vi "Shortest Distance Relative.vi"(10 "Needed angle":dbl(knob) scale=0.0..360.0, 11 "Current Angle":dbl(knob) scale=0.0..360.0) -> (2 "Flip motors?":bool, 3 "Degrees to travel":dbl)   [LabVIEW 2011, in "Pivot Drive.lvlib"]
uses:
  Pivot Drive.lvlib
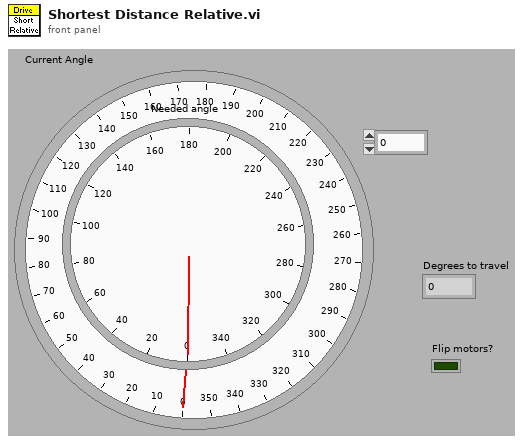
[diagram p1: front panel]
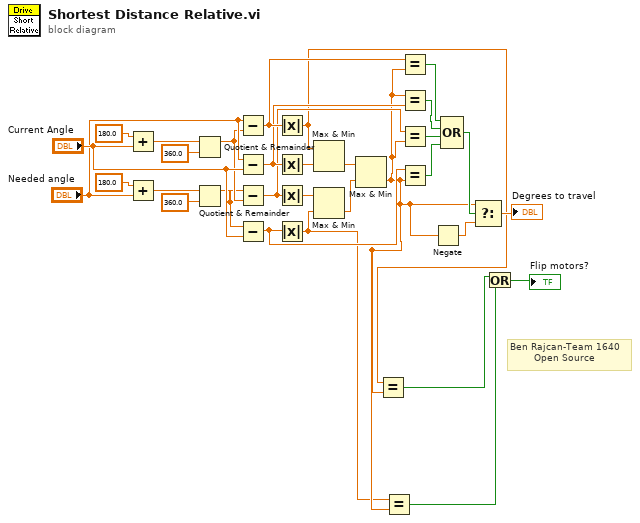
[diagram p0: block diagram]
diagram:
  # "Ben Rajcan-Team 1640\n        Open Source"
  n1 = Add(x=180.0, y="Current Angle") -> (x+y=w24:dbl)
  n2 = Add(x=180.0, y="Needed angle") -> (x+y=w27:dbl)
  n3 = Quotient & Remainder(x=w24, y=360.0) -> (x-y*floor(x/y)=w23:dbl)  [unwired: 1 out]
  n4 = Quotient & Remainder(x=w27, y=360.0) -> (x-y*floor(x/y)=w16:dbl)  [unwired: 1 out]
  n5 = Subtract(x="Needed angle", y=w23) -> (x-y=w11:dbl)
  n6 = Subtract(x="Needed angle", y="Current Angle") -> (x-y=w10:dbl)
  n7 = Subtract(x=w16, y=w23) -> (x-y=w9:dbl)
  n8 = Subtract(x=w16, y="Current Angle") -> (x-y=w8:dbl)
  n9 = Absolute Value(x=w11) -> (abs(x)=w4:dbl)
  n10 = Absolute Value(x=w10) -> (abs(x)=w3:dbl)
  n11 = Absolute Value(x=w9) -> (abs(x)=w2:dbl)
  n12 = Absolute Value(x=w8) -> (abs(x)=w1:dbl)
  n13 = Max & Min(x=w4, y=w3) -> (min(x,y)=w21:dbl)  [unwired: 1 out]
  n14 = Max & Min(x=w2, y=w1) -> (min(x,y)=w22:dbl)  [unwired: 1 out]
  n15 = Max & Min(x=w21, y=w22) -> (min(x,y)=w7:dbl)  [unwired: 1 out]
  n16 = Equal?(x=w4, y=w7) -> (x = y?=w6:bool)
  n17 = Equal?(x=w1, y=w7) -> (x = y?=w5:bool)
  n18 = Equal?(x=w11, y=w7) -> (x = y?=w12:bool)
  n19 = Equal?(x=w7, y=w10) -> (x = y?=w17:bool)
  n20 = Equal?(x=w9, y=w7) -> (x = y?=w15:bool)
  n21 = Equal?(x=w8, y=w7) -> (x = y?=w13:bool)
  n22 = Negate(x=w7) -> (-x=w18:dbl)
  n23 = Compound Arithmetic op=OR(w12, w17, w15, w13) -> (w20:bool)
  n24 = Select(t=w7, s=w20, f=w18) -> (s? t:f=→"Degrees to travel":dbl)
  n25 = Or(x=w6, y=w5) -> (x .or. y?=→"Flip motors?":bool)
